vi "PAN_AnaResp.vi"(5 "nodeID":string, 7 "add id":bool, 10 "resp in":string[](array[string])) -> (2 "resp out":string)   [LabVIEW 2016]
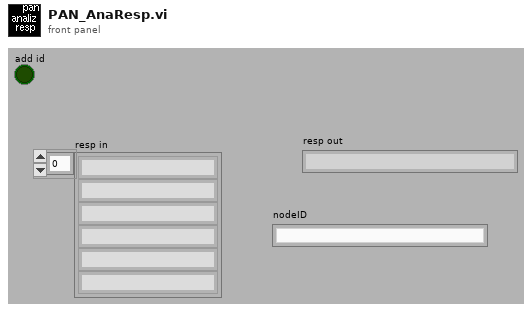
[diagram p1: front panel]
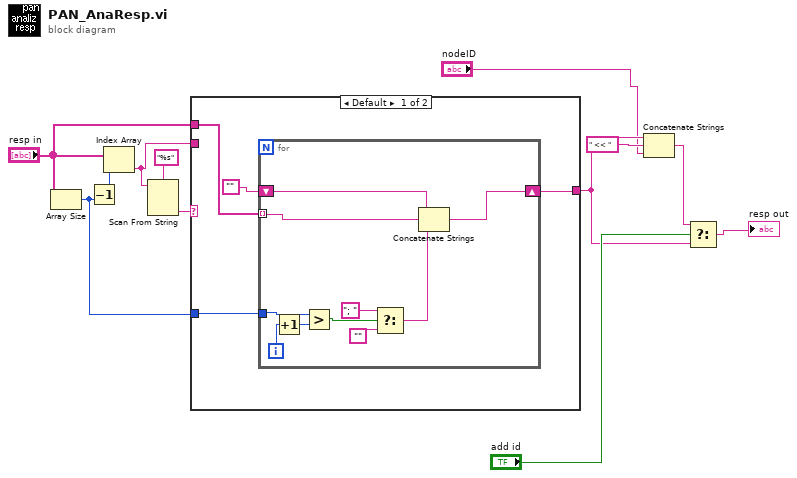
[diagram p0: block diagram]
diagram:
  n1 = Array Size(array="resp in") -> (size(s)=w7:i32)
  n2 = Decrement(x=w7) -> (x-1=w8:i32)
  n3 = Index Array(array="resp in", index=w8) -> (element=w9:string)
  n4 = Scan From String(format string="%s", input string=w9) -> (output 1=w11:string)  [unwired: 2 in, 4 out]
  n5 = case shown="Default" w11 {
    tunnel: "resp in" -> [w16 _]
    tunnel: w9 -> [_ w27]
    tunnel: [w14 w27] -> w5
    tunnel: w7 -> [w15 _]
    frame Default {
      n6 = for {
        tunnel: w16 -> [w24] mode=indexing
        shift-right: [w26] -> w14
        shift-left: "" -> [w25]
        tunnel: w15 -> [w23]
        i -> [w22]
        n7 = Increment(x=w22) -> (x+1=w18:i32)
        n8 = Greater?(x=w23, y=w18) -> (0:w21:bool)
        n9 = Select(t="; ", s=w21, f="") -> (s? t:f=w19:string)
        n10 = Concatenate Strings(w25, w24, w19) -> (w26:string)
      }
    }
    frame "OK" {
    }
  }
  n11 = Concatenate Strings(w5, " << " ("string"), "nodeID") -> (w2:string)
  n12 = Select(t=w2, s="add id", f=w5) -> (s? t:f=→"resp out":string)
